vi "Request Asynchronous Message.vi"(5 "Return Priority (Normal)":T1=enum."Normal", 6 "SubscriptionPolicy":refnum<class "ISubscriptionPolicy.lvclass">, 7 "Desired Notification Msg":refnum<class "Notification Msg.lvclass">, 8 "error in (no error)":errorcluster, 9 "Data Type":variant, 10 "Datum Name":string, 11 "IModel in":refnum<class "IModel.lvclass">) -> (0 "error out":errorcluster, 3 "IModel out":refnum<class "IModel.lvclass">)   [LabVIEW 2015, in "IModel.lvlib" / "IModel.lvclass"]
uses:
  IModel.lvclass
  IMediator/ISubscriptionPolicy/ISubscriptionPolicy.lvclass
  Transport/ActorMessage/Notification Msg/Notification Msg.lvclass
  <vilib>/ActorFramework/Message Enqueuer/Message Priority.ctl
  <vilib>/ActorFramework/Actor/Actor.lvclass/Actor.ctl
  <vilib>/ActorFramework/Message Enqueuer/Message Enqueuer.lvclass/Message Enqueuer.ctl
  IModel.lvclass/IModel.ctl
  AbstractMessages/PreAddressedMsg/PreAddressedMsg.lvclass/PreAddressedMsg.ctl
  IMediator/IMediator Messages/Subscribe Msg/Subscribe Msg.lvclass/Subscribe Msg.ctl
  <vilib>/ActorFramework/Message Enqueuer/Init from Existing Queue.vi
  <vilib>/ActorFramework/Message Enqueuer/Enqueue.vi
  AbstractMessages/PreAddressedMsg/Read Return Address.vi
  <vilib>/ActorFramework/Message Priority Queue/Priority Enqueue.vi
  <vilib>/ActorFramework/Message Enqueuer/Message Enqueuer.lvclass
  Transport/ActorMessage/ActorMessage.lvclass
  <vilib>/ActorFramework/Actor/Actor.lvclass
  IMediator/IMediator Messages/Subscribe Msg/Subscribe Msg.lvclass
  IMediator/SubscriptionRequest/SubscriptionRequest.lvclass
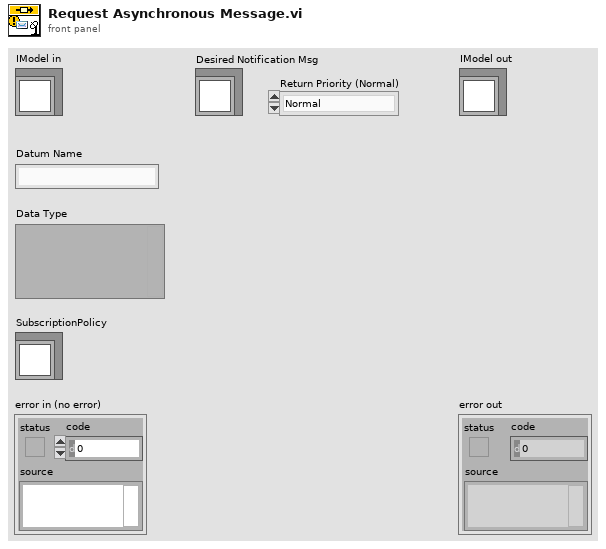
[diagram p1: front panel]
types:
  T1 = typedef "Actor Framework.lvlib/Message Enqueuer.lvclass/Message Priority.ctl" = enum16{"Low", "Normal", "High"}
  T2 = typedef "IMediator.lvlib/ISubscriptionPolicy.lvclass/ISubscriptionPolicy Reference.ctl" = refnum<data-value>
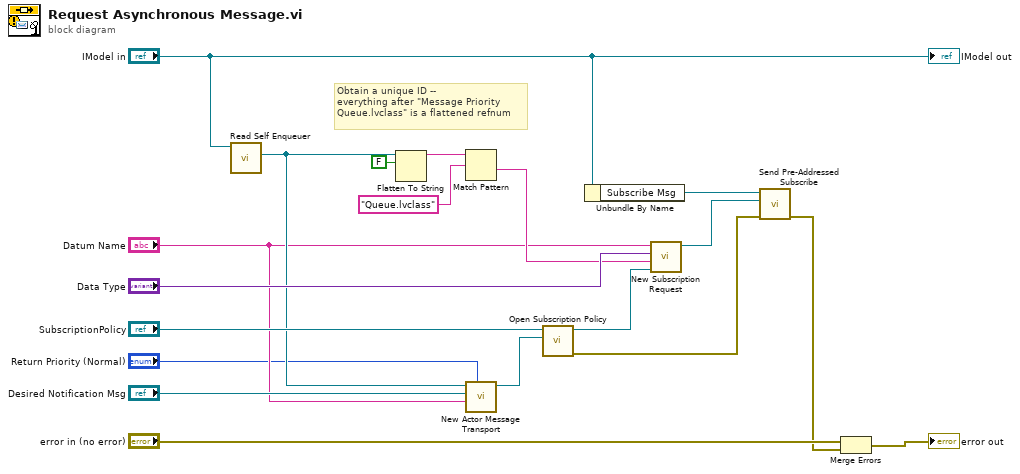
[diagram p0: block diagram]
diagram:
  # "Obtain a unique ID --\neverything after \"Message Priority\nQueue.lvclass\" is a flattened refnum"
  n1 = call <vilib>:"Read Self Enqueuer.vi"("Actor"="IModel in") -> ("Self Enqueuer"=w4:refnum<class "Message Enqueuer.lvclass">)  [unwired: 10 in]
  n2 = Flatten To String(anything=w4, prepend array or string size? (T)=FALSE) -> (data string=w11:string)  [unwired: 2 in, 2 out]
  n3 = Match Pattern(string=w11, regular expression="Queue.lvclass") -> (after substring=w8:string)  [unwired: 1 in, 3 out]
  n4 = call "New Actor Message Transport.vi"("Return Priority (Normal)"="Return Priority (Normal)", "Datum Name"="Datum Name", "Desired Notification Msg (Type)"="Desired Notification Msg", "Message Enqueuer in"=w4) -> ("ActorMessage out"=w17:refnum<class "ActorMessage.lvclass">)  [unwired: 6 in, 1 out]
  n5 = call "Open Subscription Policy.vi"("Transport"=w17, "SubscriptionPolicy"="SubscriptionPolicy") -> ("error out"=w7:errorcluster, "Subscription Policy"=w12:T2)  [unwired: 8 in]
  n6 = Unbundle By Name("IModel in") -> ("Subscribe Msg"=w15:refnum<class "Subscribe Msg.lvclass">)
  n7 = call "New Subscription Request.vi"("Subscription Policy"=w12, "Unique Subscriber ID"=w8, "Type"="Data Type", "Datum Name"="Datum Name") -> ("SubscriptionRequest"=w14:refnum<class "SubscriptionRequest.lvclass">)  [unwired: 7 in]
  n8 = call "Send Pre-Addressed Subscribe.vi"("error in (no error)"=w7, "Subscription Request"=w14, "Subscribe Msg"=w15) -> ("error out"=w5:errorcluster)  [unwired: 8 in]
  n9 = Merge Errors("error in (no error)", w5) -> (→"error out":errorcluster)
  "IModel out" <- "IModel in"
